vi "Test Run.vi"(0 "reference in":refnum<class "Test.lvclass">, 5 "error in (no error)":errorcluster) -> (14 "reference out":refnum<class "Test.lvclass">, 19 "error out":errorcluster)   [LabVIEW 2013, in "Test.lvclass"]
uses:
  Test.lvclass
  Device_class/Device.lvclass
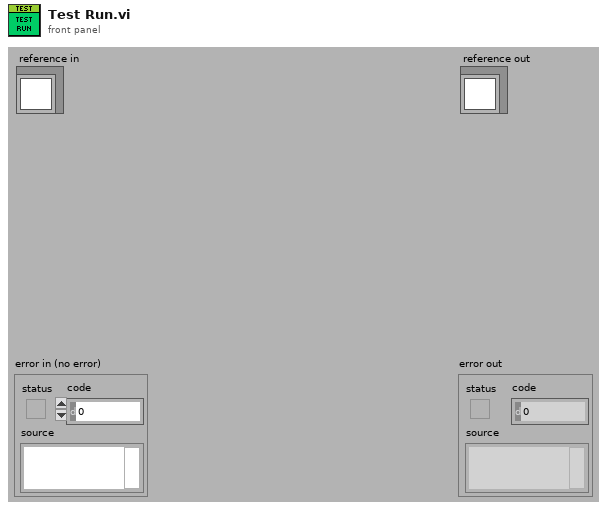
[diagram p1: front panel]
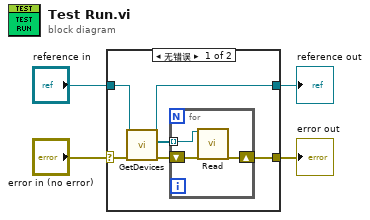
[diagram p0: block diagram]
diagram:
  n1 = case shown="无错误" "error in (no error)" {
    selector: "error in (no error)" -> [w8 w15]
    tunnel: [w10 w15] -> w3
    tunnel: [w5 w14] -> w1
    tunnel: "reference in" -> [w9 w14]
    frame No Error {
      n2 = call-dynamic "GetDevices.vi"("error in (no error)"=w8, "reference in"=w9) -> ("error out"=w7:errorcluster, "Devices"=w6:refnum<class "Device.lvclass">[], "reference out"=w5:refnum<class "Test.lvclass">)  [unwired: 7 in]
      n3 = for {
        tunnel: w6 -> [w13] mode=indexing
        shift-right: [w11] -> w10
        shift-left: w7 -> [w12]
        n4 = call-dynamic "Read.vi"("reference in"=w13, "error in (no error)"=w12) -> ("error out"=w11:errorcluster)  [unwired: 16 in, 1 out]
      }
    }
    frame Error {
    }
  }
  "error out" <- w3
  "reference out" <- w1
